vi "EX9E.vi"(11 "Variables and Memory in":T1 {"GFX" format="%02x"}) -> (3 "Variables and Memory out":T1 {"GFX" format="%02x"})   [LabVIEW 2021]
uses:
  Controls/ClusterF.ctl
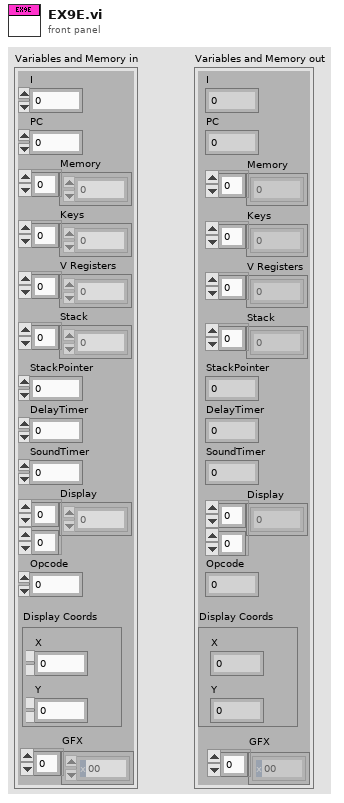
[diagram p1: front panel]
types:
  T1 = typedef "ClusterF.ctl" = cluster{"I":u16, "PC":u16, "Memory":u8[], "Keys":u8[], "V Registers":u8[], "Stack":u16[], "StackPointer":u16, "DelayTimer":u8, "SoundTimer":u8, "Display":u8[][], "Opcode":u16, "Display Coords":cluster{"X":u8, "Y":u8}, "GFX":u8[]}
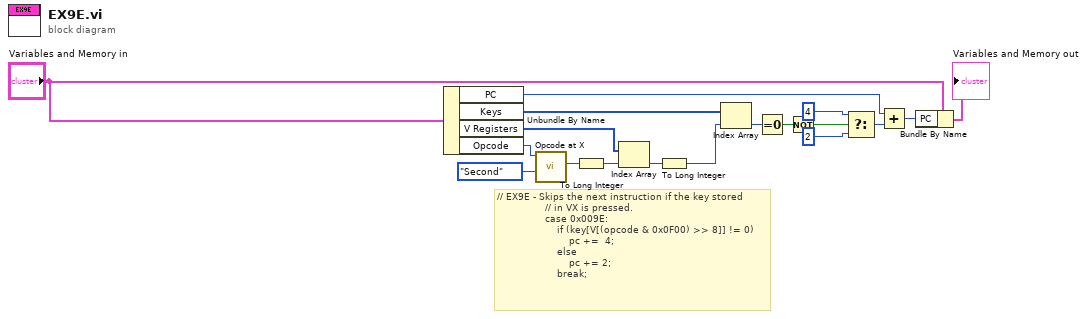
[diagram p0: block diagram]
diagram:
  # "// EX9E - Skips the next instruction if the key stored\n                // in VX is pressed.\n                case 0x009E:\n                    if (key[V[(opcode & 0x0F00) >> 8]] != 0)\n                        pc +=  4;\n                    else\n                        pc += 2;\n                    break;"
  n1 = Unbundle By Name("Variables and Memory in") -> ("PC"=w2:u16, "Keys"=w5:u8[], "V Registers"=w4:u8[], "Opcode"=w18:u16)
  n2 = call "Opcode at X.vi"("X Position"=enum16{"First", "Second", "Third", "Fourth"}."Second", "Opcode"=w18) -> ("Opcode at X Position (U8)"=w11:u8)  [unwired: 9 in]
  n3 = To Long Integer(number=w11) -> (32bit integer=w10:i32)
  n4 = Index Array(array=w4, index=w10) -> (element=w8:u8)
  n5 = To Long Integer(number=w8) -> (32bit integer=w9:i32)
  n6 = Index Array(array=w5, index=w9) -> (element=w6:u8)
  n7 = Equal To 0?(x=w6) -> (x = 0?=w7:bool)
  n8 = Not(x=w7) -> (.not. x?=w16:bool)
  n9 = Select(t=u16 4 ("y"), s=w16, f=u16 2 ("y")) -> (s? t:f=w17:u16)
  n10 = Add(x=w2, y=w17) -> (x+y=w3:u16)
  n11 = Bundle By Name(cluster="Variables and Memory in", "PC"=w3) -> (→"Variables and Memory out":T1)
